vi "ShiftRegister.vi"() -> ()   [LabVIEW 2020]
panel:
  out "Cluster":cluster{"array bool":bool[], "array num":dbl[]}
  out "Array":bool[](array[boolean])
  out "Boolean":bool
  out "concatenated string":string
  out "Numeric":i32
  in  "stop":bool
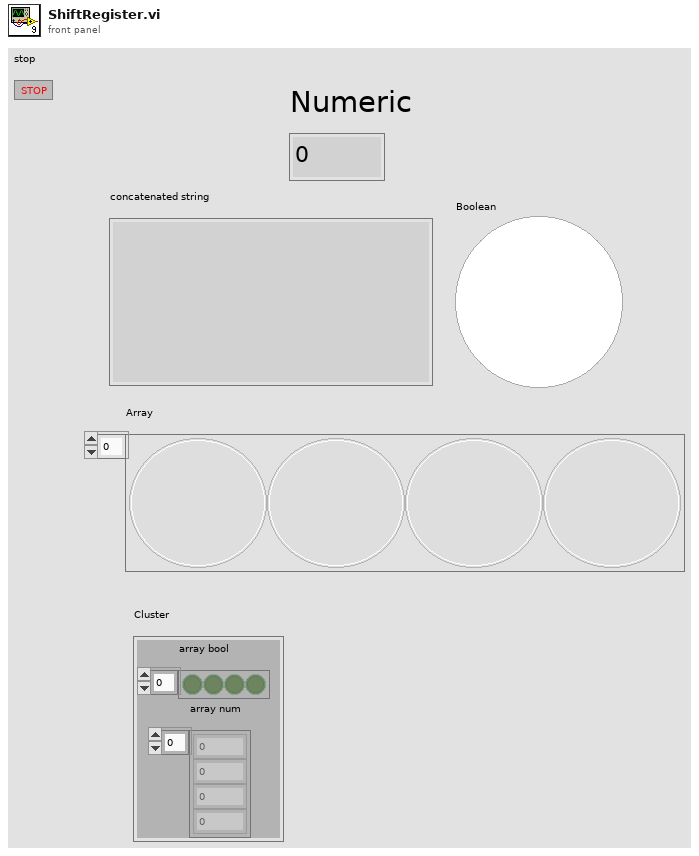
[diagram p1: front panel]
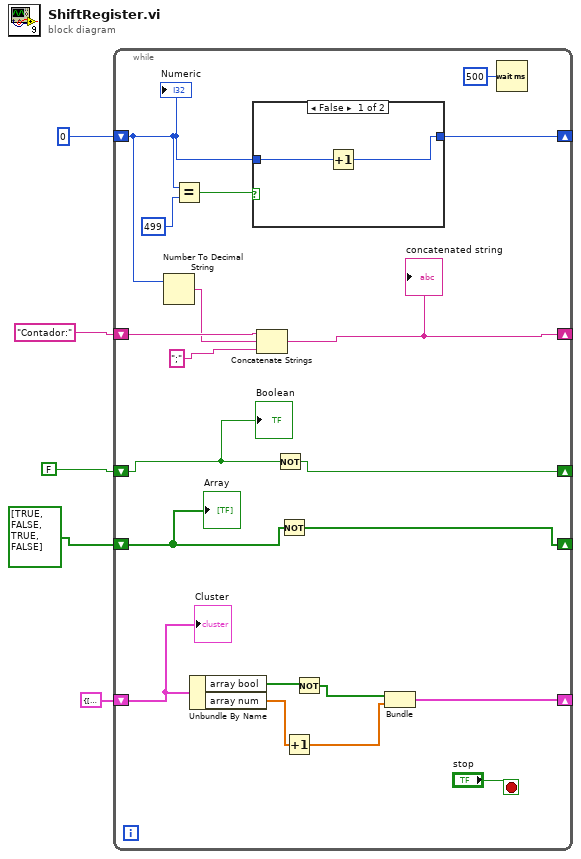
[diagram p0: block diagram]
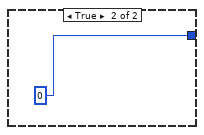
[diagram p2: hidden frame]
diagram:
  n1 = while {
    shift-right: [w22] -> _
    shift-left: 0 -> [w20]
    shift-right: [w17] -> _
    shift-left: "Contador:" -> [w19]
    shift-right: [w15] -> _
    shift-left: FALSE -> [w14]
    shift-right: [w12] -> _
    shift-left: bool[] [TRUE, FALSE, TRUE, FALSE] -> [w13]
    shift-right: [w6] -> _
    shift-left: cluster{"array bool":bool[], "array num":dbl[]} {"array bool"=[TRUE, FALSE, TRUE, FALSE], "array num"=[1.0, 2.0, 3.0, 4.0]} -> [w11]
    stop <- "stop" stop-if-true
    n2 = Number To Decimal String(number=w20) -> (decimal integer string=w18:string)  [unwired: 1 in]
    n3 = Equal?(x=w20, y=499) -> (x = y?=w24:bool)
    n4 = Unbundle By Name(w11) -> ("array bool"=w10:bool[], "array num"=w9:dbl[])
    n5 = case shown="False" w24 {
      tunnel: [w26 0] -> w22
      tunnel: w20 -> [w27 _]
      frame False {
        n6 = Increment(x=w27) -> (x+1=w26:i32)
      }
      frame True {
      }
    }
    n7 = Concatenate Strings(w19, w18, ";") -> (w17:string)
    "concatenated string" <- w17
    n8 = Not(x=w14) -> (.not. x?=w15:bool)
    n9 = Not(x=w13) -> (.not. x?=w12:bool[])
    n10 = Increment(x=w9) -> (x+1=w7:dbl[])
    n11 = Not(x=w10) -> (.not. x?=w8:bool[])
    n12 = Bundle(w8, w7) -> (w6:cluster{bool[], dbl[]})  [unwired: 1 in]
    n13 = Wait (ms)(milliseconds to wait=u32 500) -> ()  [unwired: 1 out]
    "Numeric" <- w20
    "Boolean" <- w14
    "Array" <- w13
    "Cluster" <- w11
  }
